vi "ReadConfigINI (SubVI).vi"(10 "base path":path) -> (3 "ini cluster":T1={"IP_PC"="", "IP_SNK3"="", "UDP_port_0"=0, "UDP_port_1"=0, "Serial_Code"="", "ADCToVoltage0"=0.0, "DelayChN"=[], "GainCorrection"=[[0.0, 1.0, 2.0, 3.0, 4.0, 5.0, 6.0, 7.0, 8.0, 9.0, 10.0, 11.0, 12.0, 13.0, 14.0, 15.0, 16.0, 17.0, 18.0, 19.0, 20.0, 21.0, 22.0, 23.0, 24.0, 25.0, 26.0, 27.0, 28.0, 29.0, 30.0, 31.0, 32.0, 33.0, 34.0, 35.0, 36.0, 37.0, 38.0, 39.0, 40.0], [0.007480379377256454, 0.05961025727668039, -0.2256445449069899, -0.08477459513390878, -0.19260677802883944, -0.022395839150075085, -0.076115384746043, -0.07452129161654766, -0.012380415371210218, 0.012737541388962995, 0.06895372697540661, 0.015013157866332921, -0.007045606467342559, -0.029720988817163698, 0.012859755243868034, 0.014783052645341199, 0.008698262907434648, -0.0007780407280235585, 0.0004171488690068028, 0.02092967406906331, 0.0018566195042745877, 0.009729465944000381, 0.007879136597780506, 0.028348095755020803, 0.01788279432686344, 0.01316889208220224, 0.008960543359635798, 0.01306464703510712, 0.03262709696783729, 0.0012714692473612531, -0.03761892820570949, -0.0316523389742032, 0.008159355326511571, 0.0081809109877908, 0.03836815904439456, 0.06681584703351648, 0.06544874790085742, 0.08623523673581365, 0.06010176834536063, 0.06195241245042141, 0.05245036073698361], [0.0, 0.0, 0.0, 0.0, 0.0, 0.0, 0.0, 0.0, 0.0, 0.0, 0.0, 0.0, 0.0, 0.0, 0.0, 0.0, 0.0, 0.0, 0.0, 0.0, 0.0, 0.0, 0.0, 0.0, 0.0, 0.0, 0.0, 0.0, 0.0, 0.0, 0.0, 0.0, 0.0, 0.0, 0.0, 0.0, 0.0, 0.0, 0.0, 0.0, 0.0]], "CorCh"=[], "PulseCor"=[[0.0, 1.0, 2.0, 3.0, 4.0, 5.0, 6.0, 7.0, 8.0, 9.0, 10.0, 11.0, 12.0, 13.0, 14.0, 15.0, 16.0, 17.0, 18.0, 19.0, 20.0, 21.0, 22.0, 23.0, 24.0, 25.0, 26.0, 27.0, 28.0, 29.0, 30.0, 31.0, 32.0, 33.0, 34.0, 35.0, 36.0, 37.0, 38.0, 39.0, 40.0], [0.007480379377256454, 0.05961025727668039, -0.2256445449069899, -0.08477459513390878, -0.19260677802883944, -0.022395839150075085, -0.076115384746043, -0.07452129161654766, -0.012380415371210218, 0.012737541388962995, 0.06895372697540661, 0.015013157866332921, -0.007045606467342559, -0.029720988817163698, 0.012859755243868034, 0.014783052645341199, 0.008698262907434648, -0.0007780407280235585, 0.0004171488690068028, 0.02092967406906331, 0.0018566195042745877, 0.009729465944000381, 0.007879136597780506, 0.028348095755020803, 0.01788279432686344, 0.01316889208220224, 0.008960543359635798, 0.01306464703510712, 0.03262709696783729, 0.0012714692473612531, -0.03761892820570949, -0.0316523389742032, 0.008159355326511571, 0.0081809109877908, 0.03836815904439456, 0.06681584703351648, 0.06544874790085742, 0.08623523673581365, 0.06010176834536063, 0.06195241245042141, 0.05245036073698361], [0.0, 0.0, 0.0, 0.0, 0.0, 0.0, 0.0, 0.0, 0.0, 0.0, 0.0, 0.0, 0.0, 0.0, 0.0, 0.0, 0.0, 0.0, 0.0, 0.0, 0.0, 0.0, 0.0, 0.0, 0.0, 0.0, 0.0, 0.0, 0.0, 0.0, 0.0, 0.0, 0.0, 0.0, 0.0, 0.0, 0.0, 0.0, 0.0, 0.0, 0.0]], "ADCToVoltage1"=0.0})   [LabVIEW 2017]
uses:
  Control_EU/ConfigINI.ctl
  <vilib>/Utility/config.llb/Read Key (Double).vi
  <vilib>/Utility/config.llb/Read Key (U32).vi
  <vilib>/Utility/config.llb/Read Key (String).vi
  <vilib>/Utility/config.llb/NI_LVConfig.lvlib
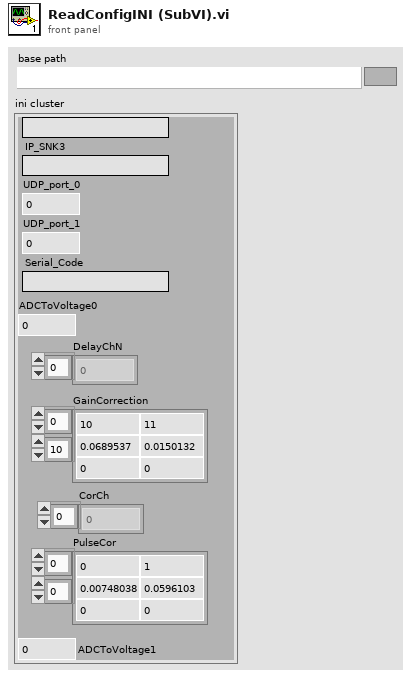
[diagram p1: front panel]
types:
  T1 = typedef "ConfigINI.ctl" = cluster{"IP_PC":string, "IP_SNK3":string, "UDP_port_0":u32, "UDP_port_1":u32, "Serial_Code":string, "ADCToVoltage0":dbl, "DelayChN":dbl[], "GainCorrection":dbl[][], "CorCh":dbl[], "PulseCor":dbl[][], "ADCToVoltage1":dbl}
  T2 = typedef "NI_LVConfig.lvlib/Config Data RefNum.ctl" = refnum<k1>
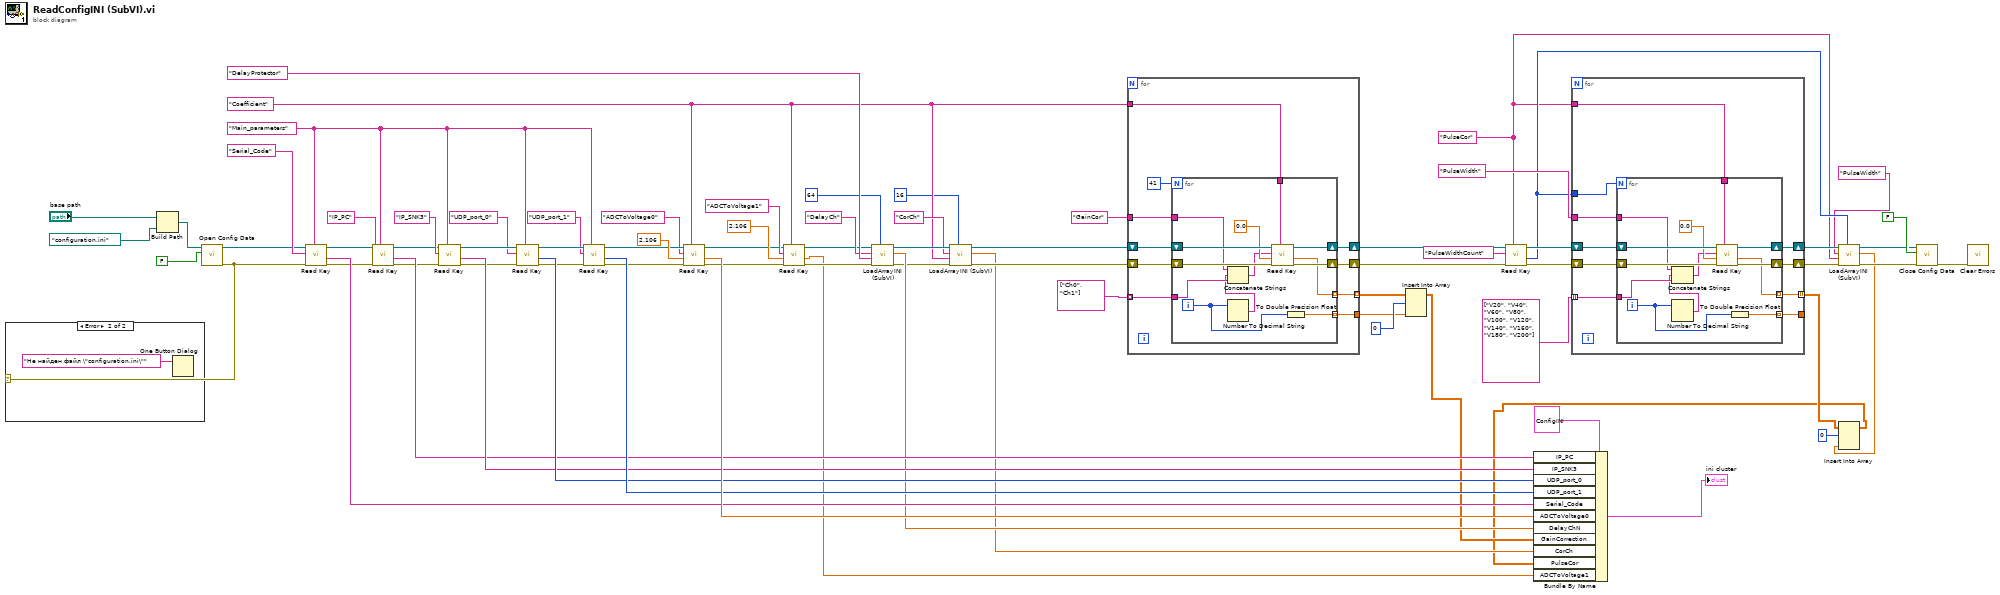
[diagram p0: block diagram]
diagram:
  w15 = "PulseCor" ("section")
  w3 = "Coefficient" ("section")
  w63 = "Main_parameters" ("section")
  n1 = Build Path(base path="base path", name or relative path=path "configuration.ini" ("default name")) -> (appended path=w52:path)
  n2 = call <vilib>:"Open Config Data.vi"("create file if necessary (T)"=FALSE ("create file if necessary? (T)"), "configuration file path"=w52) -> ("error out"=w68:errorcluster, "refnum"=w53:T2)  [unwired: 7 in, 1 out]
  n3 = case shown="Error" w68 {
    frame No Error {
    }
    frame Error {
      n4 = One Button Dialog(message="Не найден файл \"configuration.ini\"") -> ()  [unwired: 1 in, 1 out]
    }
  }
  n5 = call-poly <vilib>:"Read Key.vi"("section"=w63, "error in (no error)"=w68, "key"="Serial_Code", "refnum"=w53) -> ("error out"=w56:errorcluster, "value"=w76:string, "refnum out"=w55:T2)  [unwired: 4 in, 1 out]
  n6 = call-poly <vilib>:"Read Key.vi"("section"=w63, "error in (no error)"=w56, "key"="IP_PC", "refnum"=w55) -> ("error out"=w59:errorcluster, "value"=w72:string, "refnum out"=w58:T2)  [unwired: 4 in, 1 out]
  n7 = call-poly <vilib>:"Read Key.vi"("section"=w63, "error in (no error)"=w59, "key"="IP_SNK3", "refnum"=w58) -> ("error out"=w65:errorcluster, "value"=w73:string, "refnum out"=w67:T2)  [unwired: 4 in, 1 out]
  n8 = call-poly <vilib>:"Read Key.vi"("section"=w63, "error in (no error)"=w65, "key"="UDP_port_0", "refnum"=w67) -> ("error out"=w64:errorcluster, "value"=w74:u32, "refnum out"=w66:T2)  [unwired: 4 in, 1 out]
  n9 = call-poly <vilib>:"Read Key.vi"("section"=w63, "error in (no error)"=w64, "key"="UDP_port_1", "refnum"=w66) -> ("error out"=w35:errorcluster, "value"=w75:u32, "refnum out"=w70:T2)  [unwired: 4 in, 1 out]
  n10 = call-poly <vilib>:"Read Key.vi"("section"=w3, "error in (no error)"=w35, "default value"=2.106, "key"="ADCToVoltage0", "refnum"=w70) -> ("error out"=w5:errorcluster, "value"=w77:dbl, "refnum out"=w6:T2)  [unwired: 3 in, 1 out]
  n11 = call-poly <vilib>:"Read Key.vi"("section"=w3, "error in (no error)"=w5, "default value"=2.106, "key"="ADCToVoltage1", "refnum"=w6) -> ("error out"=w4:errorcluster, "value"=w2:dbl, "refnum out"=w7:T2)  [unwired: 3 in, 1 out]
  n12 = call "LoadArrayINI (SubVI).vi"("Numeric"=64, "error in (no error)"=w4, "section"="DelayProtector", "key"="DelayCh", "Refnum in"=w7) -> ("error out"=w34:errorcluster, "Array"=w43:dbl[], "Refnum out"=w33:T2)  [unwired: 4 in]
  n13 = call "LoadArrayINI (SubVI).vi"("Numeric"=16, "error in (no error)"=w34, "section"=w3, "key"="CorCh", "Refnum in"=w33) -> ("error out"=w31:errorcluster, "Array"=w28:dbl[], "Refnum out"=w32:T2)  [unwired: 4 in]
  n14 = for {
    tunnel: w3 -> [w87]
    tunnel: string[] ["Ch0", "Ch1"] -> [w86] mode=indexing
    tunnel: [w85] -> w41 mode=indexing
    shift-right: [w82] -> w27
    shift-left: w32 -> [w84]
    shift-right: [w81] -> w26
    shift-left: w31 -> [w83]
    tunnel: [w80] -> w38
    tunnel: "GainCor" ("key") -> [w79]
    n15 = for {
      N: 41 -> [_]
      tunnel: w87 -> [w96]
      shift-right: [w98] -> w82
      shift-left: w84 -> [w101]
      shift-right: [w99] -> w81
      shift-left: w83 -> [w100]
      tunnel: [w95] -> w85 mode=indexing
      tunnel: w86 -> [w93]
      tunnel: [w90] -> w80 mode=indexing
      tunnel: w79 -> [w89]
      i -> [w91]
      n16 = Number To Decimal String(number=w91) -> (decimal integer string=w92:string)  [unwired: 1 in]
      n17 = Concatenate Strings(w89, w92, w93) -> (w94:string)
      n18 = call-poly <vilib>:"Read Key.vi"("section"=w96, "error in (no error)"=w100, "default value"=0.0, "key"=w94, "refnum"=w101) -> ("error out"=w99:errorcluster, "value"=w95:dbl, "refnum out"=w98:T2)  [unwired: 3 in, 1 out]
      n19 = To Double Precision Float(number=w91) -> (double precision float=w90:dbl)
    }
  }
  n20 = Insert Into Array(array=w41, index (row)=0, new element=w38) -> (w39:dbl[][])  [unwired: 1 in]
  n21 = call-poly <vilib>:"Read Key.vi"("section"=w15, "error in (no error)"=w26, "key"="PulseWidthCount", "refnum"=w27) -> ("error out"=w23:errorcluster, "value"=w16:u32, "refnum out"=w24:T2)  [unwired: 4 in, 1 out]
  n22 = for {
    tunnel: w15 -> [w111]
    tunnel: string[] ["V20", "V40", "V60", "V80", "V100", "V120", "V140", "V160", "V180", "V200"] -> [w110] mode=indexing
    tunnel: [w109] -> w13 mode=indexing
    shift-right: [w106] -> w20
    shift-left: w24 -> [w108]
    shift-right: [w105] -> w18
    shift-left: w23 -> [w107]
    tunnel: [w104] -> _
    tunnel: "PulseWidth" ("section") -> [w103]
    tunnel: w16 -> [w102]
    n23 = for {
      N: w102 -> [_]
      tunnel: w111 -> [w119]
      shift-right: [w121] -> w106
      shift-left: w108 -> [w124]
      shift-right: [w122] -> w105
      shift-left: w107 -> [w123]
      tunnel: [w118] -> w109 mode=indexing
      tunnel: w110 -> [w116]
      tunnel: [w113] -> w104 mode=indexing
      tunnel: w103 -> [w112]
      i -> [w114]
      n24 = Number To Decimal String(number=w114) -> (decimal integer string=w115:string)  [unwired: 1 in]
      n25 = Concatenate Strings(w112, w115, w116) -> (w117:string)
      n26 = call-poly <vilib>:"Read Key.vi"("section"=w119, "error in (no error)"=w123, "default value"=0.0, "key"=w117, "refnum"=w124) -> ("error out"=w122:errorcluster, "value"=w118:dbl, "refnum out"=w121:T2)  [unwired: 3 in, 1 out]
      n27 = To Double Precision Float(number=w114) -> (double precision float=w113:dbl)
    }
  }
  n28 = call "LoadArrayINI (SubVI).vi"("Numeric"=w16, "error in (no error)"=w18, "section"=w15, "key"="PulseWidth" ("section"), "Refnum in"=w20) -> ("error out"=w17:errorcluster, "Array"=w12:dbl[], "Refnum out"=w19:T2)  [unwired: 4 in]
  n29 = Insert Into Array(array=w13, index (row)=0, new element=w12) -> (w10:dbl[][])  [unwired: 1 in]
  n30 = Bundle By Name(cluster=T1 {"IP_PC"="", "IP_SNK3"="", "UDP_port_0"=0, "UDP_port_1"=0, "Serial_Code"="", "ADCToVoltage0"=0.0, "DelayChN"=[], "GainCorrection"=[[0.0, 1.0, 2.0, 3.0, 4.0, 5.0, 6.0, 7.0, 8.0, 9.0, 10.0, 11.0, 12.0, 13.0, 14.0, 15.0, 16.0, 17.0, 18.0, 19.0, 20.0, 21.0, 22.0, 23.0, 24.0, 25.0, 26.0, 27.0, 28.0, 29.0, 30.0, 31.0, 32.0, 33.0, 34.0, 35.0, 36.0, 37.0, 38.0, 39.0, 40.0], [0.007480379377256454, 0.05961025727668039, -0.2256445449069899, -0.08477459513390878, -0.19260677802883944, -0.022395839150075085, -0.076115384746043, -0.07452129161654766, -0.012380415371210218, 0.012737541388962995, 0.06895372697540661, 0.015013157866332921, -0.007045606467342559, -0.029720988817163698, 0.012859755243868034, 0.014783052645341199, 0.008698262907434648, -0.0007780407280235585, 0.0004171488690068028, 0.02092967406906331, 0.0018566195042745877, 0.009729465944000381, 0.007879136597780506, 0.028348095755020803, 0.01788279432686344, 0.01316889208220224, 0.008960543359635798, 0.01306464703510712, 0.03262709696783729, 0.0012714692473612531, -0.03761892820570949, -0.0316523389742032, 0.008159355326511571, 0.0081809109877908, 0.03836815904439456, 0.06681584703351648, 0.06544874790085742, 0.08623523673581365, 0.06010176834536063, 0.06195241245042141, 0.05245036073698361], [0.0, 0.0, 0.0, 0.0, 0.0, 0.0, 0.0, 0.0, 0.0, 0.0, 0.0, 0.0, 0.0, 0.0, 0.0, 0.0, 0.0, 0.0, 0.0, 0.0, 0.0, 0.0, 0.0, 0.0, 0.0, 0.0, 0.0, 0.0, 0.0, 0.0, 0.0, 0.0, 0.0, 0.0, 0.0, 0.0, 0.0, 0.0, 0.0, 0.0, 0.0]], "CorCh"=[], "PulseCor"=[[0.0, 1.0, 2.0, 3.0, 4.0, 5.0, 6.0, 7.0, 8.0, 9.0, 10.0, 11.0, 12.0, 13.0, 14.0, 15.0, 16.0, 17.0, 18.0, 19.0, 20.0, 21.0, 22.0, 23.0, 24.0, 25.0, 26.0, 27.0, 28.0, 29.0, 30.0, 31.0, 32.0, 33.0, 34.0, 35.0, 36.0, 37.0, 38.0, 39.0, 40.0], [0.007480379377256454, 0.05961025727668039, -0.2256445449069899, -0.08477459513390878, -0.19260677802883944, -0.022395839150075085, -0.076115384746043, -0.07452129161654766, -0.012380415371210218, 0.012737541388962995, 0.06895372697540661, 0.015013157866332921, -0.007045606467342559, -0.029720988817163698, 0.012859755243868034, 0.014783052645341199, 0.008698262907434648, -0.0007780407280235585, 0.0004171488690068028, 0.02092967406906331, 0.0018566195042745877, 0.009729465944000381, 0.007879136597780506, 0.028348095755020803, 0.01788279432686344, 0.01316889208220224, 0.008960543359635798, 0.01306464703510712, 0.03262709696783729, 0.0012714692473612531, -0.03761892820570949, -0.0316523389742032, 0.008159355326511571, 0.0081809109877908, 0.03836815904439456, 0.06681584703351648, 0.06544874790085742, 0.08623523673581365, 0.06010176834536063, 0.06195241245042141, 0.05245036073698361], [0.0, 0.0, 0.0, 0.0, 0.0, 0.0, 0.0, 0.0, 0.0, 0.0, 0.0, 0.0, 0.0, 0.0, 0.0, 0.0, 0.0, 0.0, 0.0, 0.0, 0.0, 0.0, 0.0, 0.0, 0.0, 0.0, 0.0, 0.0, 0.0, 0.0, 0.0, 0.0, 0.0, 0.0, 0.0, 0.0, 0.0, 0.0, 0.0, 0.0, 0.0]], "ADCToVoltage1"=0.0} ("Value"), "IP_PC"=w72, "IP_SNK3"=w73, "UDP_port_0"=w74, "UDP_port_1"=w75, "Serial_Code"=w76, "ADCToVoltage0"=w77, "DelayChN"=w43, "GainCorrection"=w39, "CorCh"=w28, "PulseCor"=w10, "ADCToVoltage1"=w2) -> (→"ini cluster":T1)
  n31 = call <vilib>:"Close Config Data.vi"("error in (no error)"=w17, "write file if changed (T)"=FALSE ("write configuration file? (T)"), "refnum"=w19) -> ("error out"=w50:errorcluster)  [unwired: 8 out]
  n32 = call <vilib>:"Clear Errors.vi"("error in (no error)"=w50) -> ()  [unwired: 5 in, 2 out]
